vi "Create Cal Stimulus.vi"(8 "error in (no error)":errorcluster, 11 "Cal Stimulus":T1={"Min Freq (Hz)"=50.0, "Max Freq (Hz)"=50000.0, "Freq Step (Hz)"=50.0, "Waveform"=enum."Chirp", "Attenuation (dB)"=20.0, "Sample Rate (Hz)"=100000.0}) -> (0 "error out":errorcluster, 2 "Stimulus waveform":cluster{i32, dbl, dbl[]}, 3 "Stimulus":dbl[](array[numeric]))   [LabVIEW 2020]
uses:
  Type Defs/Cal Stimulus.ctl
  <vilib>/Analysis/2dsp.llb/Inverse Complex FFT.vi
  <vilib>/Analysis/NI_AALPro.lvlib
panel:
  out "Phase graph":cluster{i32, "Freq Step (Hz)":dbl, dbl[]}(graph)
  out "Magnitude graph":cluster{i32, "Freq Step (Hz)":dbl, dbl[]}(graph)
  out "Signal graph":cluster{i32, dbl, dbl[]}(graph)
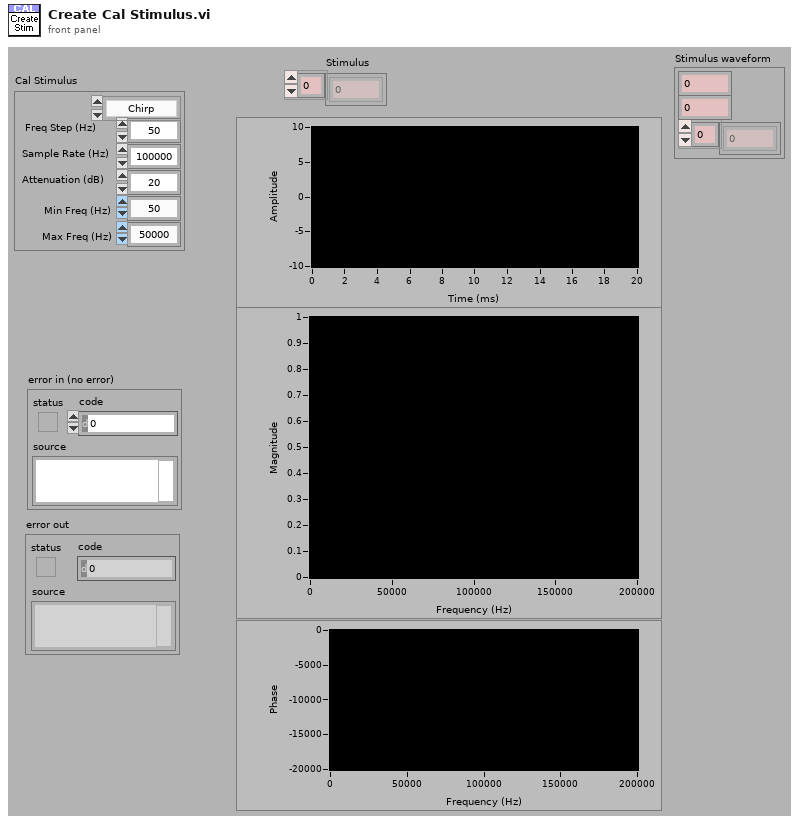
[diagram p1: front panel]
types:
  T1 = typedef "Cal Stimulus.ctl" = cluster{"Min Freq (Hz)":dbl, "Max Freq (Hz)":dbl, "Freq Step (Hz)":dbl, "Waveform":enum16{"Chirp", "Weighted"}, "Attenuation (dB)":dbl, "Sample Rate (Hz)":dbl}
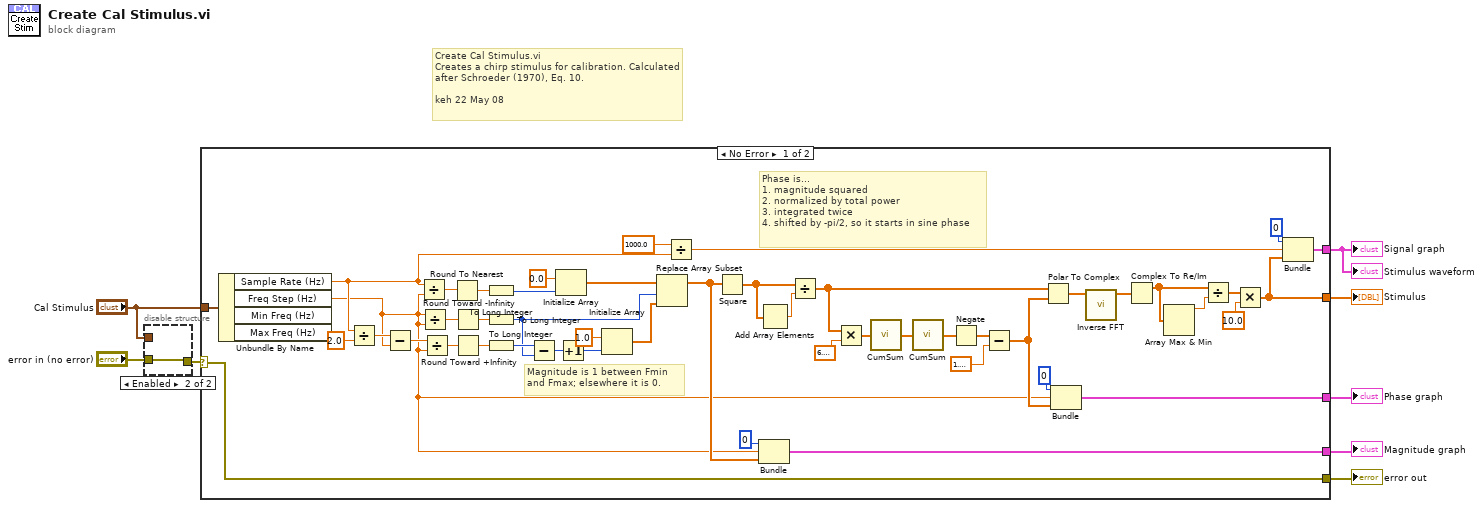
[diagram p0: block diagram]
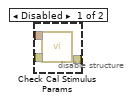
[diagram p2: hidden frame]
diagram:
  # "Create Cal Stimulus.vi\nCreates a chirp stimulus for calibration. Calculated after Schroeder (1970), Eq. 10.\n\nkeh 22 May 08"
  n1 = disable-structure shown="Enabled" {
    disable-tunnel: "Cal Stimulus" -> [w11 _]
    disable-tunnel: [w10 w12] -> w4
    disable-tunnel: "error in (no error)" -> [w9 w12]
    frame Disabled {
      n2 = call "Check Cal Stimulus Params.vi"("error in (no error)"=w9, "Cal Stimulus"=w11) -> ("error out"=w10:errorcluster)  [unwired: 9 in]
    }
    frame Enabled {
    }
  }
  n3 = case shown="No Error" w4 {
    selector: w4 -> [w21 w61]
    tunnel: "Cal Stimulus" -> [w60 _]
    tunnel: [w59 _] -> w8
    tunnel: [w58 _] -> w7
    tunnel: [w57 _] -> w6
    tunnel: [w56 _] -> w1
    tunnel: [w21 w61] -> w2
    frame No Error {
      # "Phase is...\n1. magnitude squared\n2. normalized by total power\n3. integrated twice\n4. shifted by -pi/2, so it starts in sine phase"
      # "Magnitude is 1 between Fmin\nand Fmax; elsewhere it is 0."
      n4 = Unbundle By Name(w60) -> ("Sample Rate (Hz)"=w15:dbl, "Freq Step (Hz)"=w13:dbl)  [unwired: 2 out]
      n5 = Divide(x=w15, y=2.0) -> (x/y=w16:dbl)
      n6 = Subtract(x=w16, y=w13) -> (x-y=w17:dbl)
      n7 = Divide(x=w15, y=w13) -> (x/y=w55:dbl)
      n8 = Divide(x=w13, y=w13) -> (x/y=w51:dbl)
      n9 = Divide(x=w17, y=w13) -> (x/y=w50:dbl)
      n10 = Round To Nearest(number=w55) -> (nearest integer value=w54:dbl)
      n11 = Round Toward -Infinity(1:w51) -> (0:w48:dbl)
      n12 = Round Toward +Infinity(x=w50) -> (ceil(x): smallest int >= x=w49:dbl)
      n13 = To Long Integer(number=w54) -> (32bit integer=w53:i32)
      n14 = To Long Integer(number=w48) -> (32bit integer=w44:i32)
      n15 = To Long Integer(number=w49) -> (32bit integer=w45:i32)
      n16 = Subtract(x=w45, y=w44) -> (x-y=w43:i32)
      n17 = Initialize Array(0.0 ("element"), w53) -> (w47:dbl[])
      n18 = Increment(x=w43) -> (x+1=w42:i32)
      n19 = Initialize Array(1.0 ("element"), w42) -> (w41:dbl[])
      n20 = Replace Array Subset(array=w47, new element=w41, index=w44) -> (w39:dbl[])
      n21 = Divide(x=1000.0, y=w15) -> (x/y=w23:dbl)
      n22 = Square(x=w39) -> (x^2=w38:dbl[])
      n23 = Bundle(0, "Freq Step (Hz)"=w13, w39) -> (w59:cluster{i32, "Freq Step (Hz)":dbl, dbl[]})  [unwired: 1 in]
      n24 = Add Array Elements(numeric array=w38) -> (sum=w37:dbl)
      n25 = Divide(x=w38, y=w37) -> (x/y=w31:dbl[])
      n26 = Multiply(x=w31, y=6.283185307179586) -> (x*y=w35:dbl[])
      n27 = call "CumSum.vi"("Array"=w35) -> ("CumSum"=w34:dbl[])
      n28 = call "CumSum.vi"("Array"=w34) -> ("CumSum"=w33:dbl[])
      n29 = Negate(x=w33) -> (-x=w28:dbl[])
      n30 = Subtract(x=w28, y=1.5707963267948966) -> (x-y=w27:dbl[])
      n31 = Polar To Complex(1:w27, 2:w31) -> (0:w30:cdb[])
      n32 = Bundle(0, "Freq Step (Hz)"=w13, w27) -> (w58:cluster{i32, "Freq Step (Hz)":dbl, dbl[]})  [unwired: 1 in]
      n33 = call-poly <vilib>:"Inverse FFT.vi"("FFT {X}"=w30) -> ("X"=w29:cdb[])  [unwired: 9 in, 1 out]
      n34 = Complex To Re/Im(x + iy=w29) -> (x=w22:dbl[])  [unwired: 1 out]
      n35 = Array Max & Min(array=w22) -> (max value=w20:dbl)  [unwired: 3 out]
      n36 = Divide(x=w22, y=w20) -> (x/y=w19:dbl[])
      n37 = Multiply(x=w19, y=10.0) -> (x*y=w56:dbl[])
      n38 = Bundle(0, w23, w56) -> (w57:cluster{i32, dbl, dbl[]})  [unwired: 1 in]
    }
    frame Error {
    }
  }
  "Stimulus" <- w1
  "Signal graph" <- w6
  "Magnitude graph" <- w8
  "Phase graph" <- w7
  "Stimulus waveform" <- w6
  "error out" <- w2
